vi "demo ui.vi"() -> ()   [LabVIEW 2013]
panel:
  out "Numeric 2":dbl format="%.1f"
  out "Numeric":dbl format="%.1f"
  out "Color Ramp 2":dbl(ramp)
  out "Color Ramp":dbl(ramp)
  in  "Teacher":bool
  in  "Setup":bool
  in  "Experiment":bool
  in  "MainTab":T1(tab)
  in  "SetupTab":enum32{"Page 1", "Page 2", "Page 3"}(tab)
  out "Step #":dbl
  in  "Next Button":bool
  in  "Previous Button":bool
  out "Waveform Chart 2":cluster{"Slide":dbl, "One Cube":dbl}(graph)
  out "Thermometer":dbl(slide) scale=0.0..100.0
  # "Setup"
  # "This is the myDAQ"
  # "Plug the myDAQ into the computer with a USB cable"
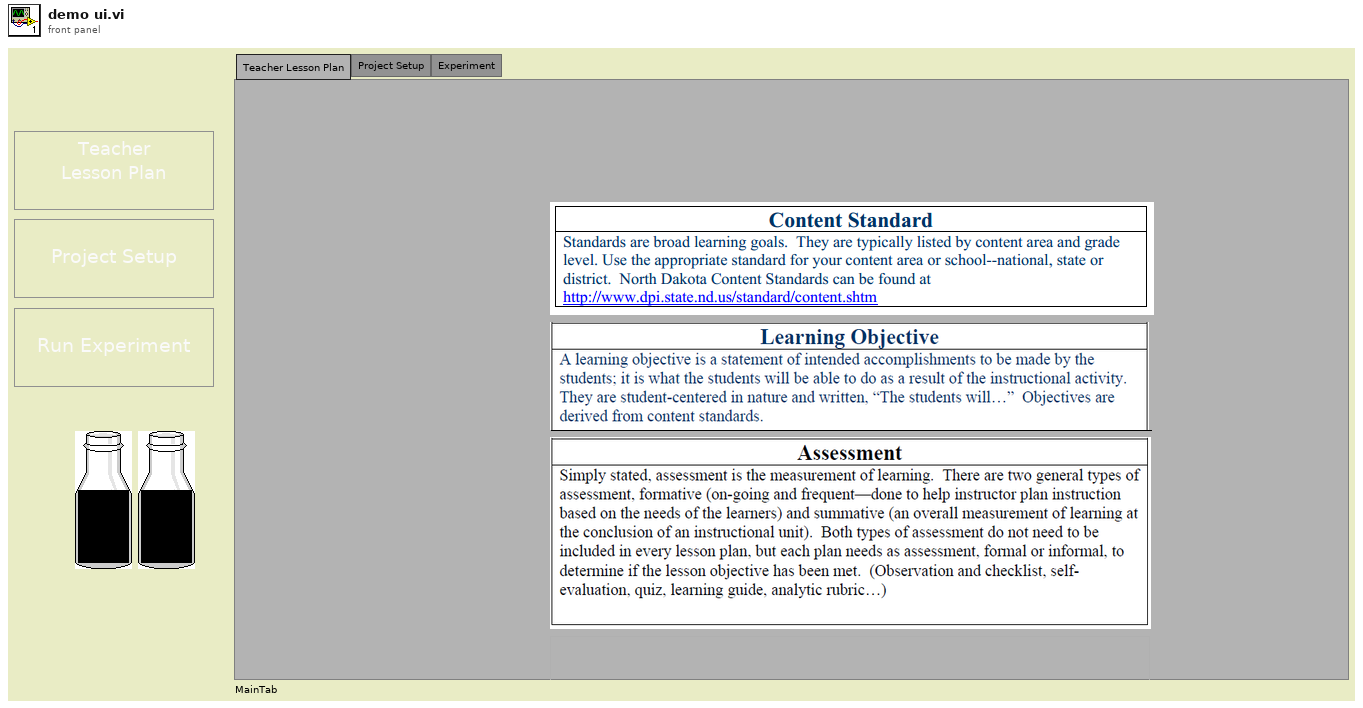
[diagram p1: front panel]
types:
  T1 = enum32{"Teacher Lesson Plan", "Project Setup", "Experiment"}
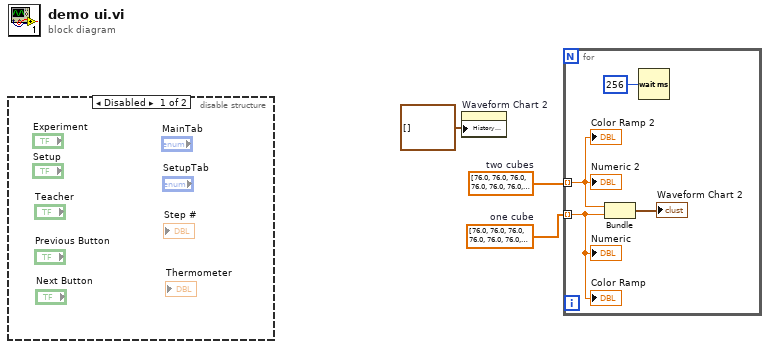
[diagram p0: block diagram]
diagram:
  w2 = dbl[] [76.0, 76.0, 76.0, 76.0, 76.0, 76.0, 76.0, 75.3529411764706, 74.49019607843138, 73.62745098039215, 72.76470588235294, 71.90196078431373, 71.03921568627452, 69.31372549019608, 68.01960784313725, 66.50980392156863, 64.7843137254902, 63.70588235294118, 62.411764705882355, 61.76470588235294, 60.90196078431373, 60.254901960784316, 59.1764705882353, 58.09803921568628, 57.01960784313726, 55.72549019607843, 54.431372549019606, 53.35294117647059, 52.05882352941177, 51.19607843137255, 50.549019607843135, 49.470588235294116, 48.6078431372549, 47.745098039215684, 46.88235294117647, 46.23529411764706, 45.588235294117645, 44.294117647058826, 43.431372549019606, 42.78431372549019, 41.490196078431374, 40.411764705882355, 39.333333333333336, 38.68627450980392, 38.254901960784316, 37.8235294117647, 37.1764705882353, 36.745098039215684, 36.529411764705884, 36.31372549019608, 35.666666666666664, 35.450980392156865, 34.80392156862745, 34.372549019607845, 34.372549019607845, 34.372549019607845, 34.15686274509804, 34.15686274509804, 34.15686274509804, 34.15686274509804, 34.15686274509804, 33.94117647058823, 33.94117647058823, 33.509803921568626, 33.509803921568626, 33.294117647058826, 33.07843137254902, 33.07843137254902, 32.86274509803921, 32.64705882352941, 32.64705882352941, 32.431372549019606, 32.431372549019606, 32.21568627450981, 32.21568627450981, 32.0, 32.0, 32.0, 32.0, 32.0, 32.0, 32.0, 32.0, 32.0, 32.0, 32.0, 32.0, 32.0, 32.0, 32.0, 32.0, 32.0, 32.0, 32.0, 32.0, 32.0, 32.0, 32.0, 32.0, 32.0, 32.0, 32.0, 32.0, 32.0, 32.0, 32.0, 32.0, 32.0, 32.0]  # two cubes
  w3 = dbl[] [76.0, 76.0, 76.0, 76.0, 76.0, 76.0, 76.0, 76.0, 76.0, 76.0, 76.0, 75.45679012345678, 75.45679012345678, 74.64197530864197, 73.82716049382717, 73.28395061728395, 72.74074074074073, 72.74074074074073, 72.74074074074073, 72.46913580246914, 71.92592592592592, 71.38271604938271, 70.8395061728395, 70.29629629629629, 70.02469135802468, 69.20987654320987, 68.39506172839506, 67.30864197530865, 66.76543209876543, 66.22222222222221, 65.67901234567901, 64.86419753086419, 63.77777777777778, 62.96296296296296, 62.148148148148145, 61.33333333333333, 60.24691358024691, 59.7037037037037, 59.432098765432094, 58.34567901234568, 57.25925925925926, 56.98765432098765, 55.901234567901234, 55.08641975308642, 54.0, 52.641975308641975, 51.82716049382716, 51.28395061728395, 50.19753086419753, 49.65432098765432, 48.839506172839506, 48.5679012345679, 47.48148148148148, 46.39506172839506, 45.58024691358025, 44.76543209876543, 43.95061728395061, 42.864197530864196, 42.32098765432099, 42.32098765432099, 42.32098765432099, 41.50617283950617, 41.50617283950617, 40.96296296296296, 40.96296296296296, 40.41975308641975, 40.41975308641975, 40.148148148148145, 39.876543209876544, 39.876543209876544, 39.876543209876544, 39.876543209876544, 39.876543209876544, 39.876543209876544, 39.876543209876544, 39.333333333333336, 39.333333333333336, 39.06172839506173, 39.06172839506173, 38.79012345679012, 38.51851851851852, 37.7037037037037, 37.4320987654321, 37.4320987654321, 37.160493827160494, 36.888888888888886, 36.888888888888886, 36.34567901234568, 36.074074074074076, 35.80246913580247, 35.53086419753087, 35.53086419753087, 34.98765432098765, 34.44444444444444, 34.44444444444444, 34.17283950617284, 33.629629629629626, 33.358024691358025, 33.08641975308642, 32.81481481481482, 32.54320987654321, 32.27160493827161, 32.0, 32.0, 32.0, 32.0, 32.0, 32.0, 32.0, 32.0, 32.0, 32.0, 32.0, 32.0, 32.0, 32.0, 32.0, 32.0, 32.0, 32.0, 32.0, 32.0, 32.0, 32.0, 32.0]  # one cube
  n1 = disable-structure shown="Disabled" {
    frame Disabled {
    }
    frame Enabled {
    }
  }
  n2 = property on="Waveform Chart 2" class="WFChart (strict)"("History Data"=cluster{"Slide":dbl, "One Cube":dbl}[] []) -> ()  [unwired: 2 in, 2 out]
  n3 = for {
    tunnel: w3 -> [w4] mode=indexing
    tunnel: w2 -> [w5] mode=indexing
    n4 = Bundle("Slide"=w5, "One Cube"=w4) -> (→"Waveform Chart 2":cluster{"Slide":dbl, "One Cube":dbl})  [unwired: 1 in]
    n5 = Wait (ms)(milliseconds to wait=u32 256) -> ()  [unwired: 1 out]
    "Color Ramp" <- w4
    "Color Ramp 2" <- w5
    "Numeric 2" <- w5
    "Numeric" <- w4
  }
